vi "_Get Loop Time (FPGA us).vi"() -> (0 "Loop Time (us)":u32)   [LabVIEW 2016]
panel:
  # "This VI returns the time difference between sucessive calls.\nUsing a feedback node without a loop was made possible in LabVIEW 8.5.  This node will always return 0 on its first call."
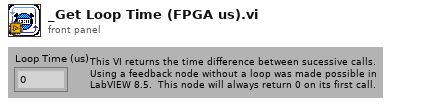
[diagram p1: front panel]
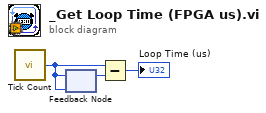
[diagram p0: block diagram]
diagram:
  n1 = call "Tick Count"() -> ("Tick Count(uSec)"=w1:u32)
  n2 = feedback-in #1(w1) -> ()
  n3 = feedback #1(w1) -> (w2:u32)
  n4 = Subtract(x=w1, y=w2) -> (x-y=→"Loop Time (us)":u32)
